vi "Launch Plugins.vi"(8 "error in":errorcluster, 11 "Master Controller in":refnum<class "EMS User Interface.lvclass">) -> (0 "error out":errorcluster, 3 "Master Controller out":refnum<class "EMS User Interface.lvclass">)   [LabVIEW 2018, in "EMS User Interface Actor.lvlib" / "EMS User Interface.lvclass"]
doc: "Launch SCADA. This nested actor handles all of the optimization and communication actors, so the Master Controller Core can focus on UI interaction."
uses:
  EMS User Interface.lvclass
  <vilib>/ActorFramework/Actor/Actor.lvclass
  EMS Generic Actor/EMS Generic/EMS Generic.lvclass
  C:/Users/Administrator/Desktop/2018LabVIEW EMS/EMS Generic Actor/EMS Generic/EMS Generic.lvclass
  C:/Program Files (x86)/National Instruments/LabVIEW 2018/vi.lib/ActorFramework/Actor/Actor.lvclass
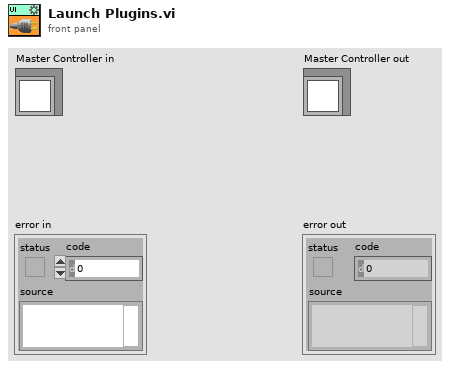
[diagram p1: front panel]
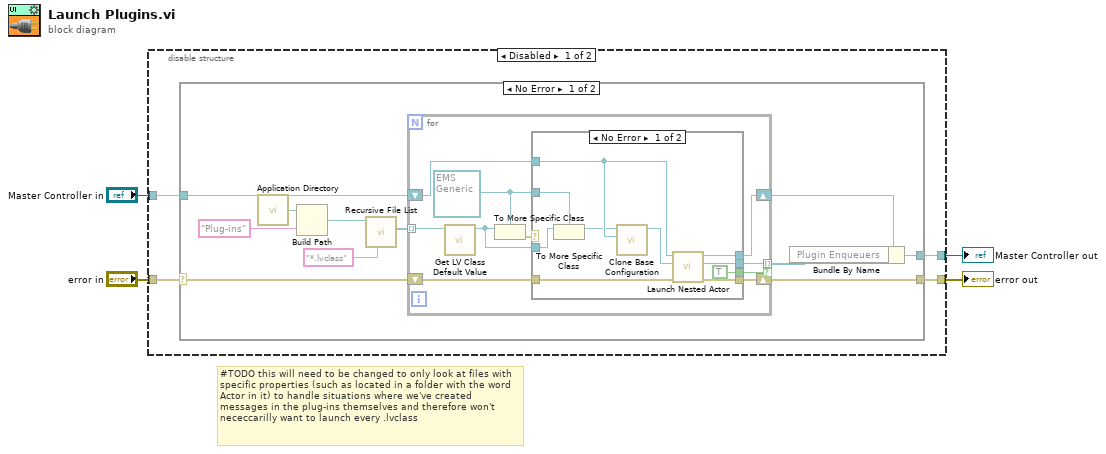
[diagram p0: block diagram]
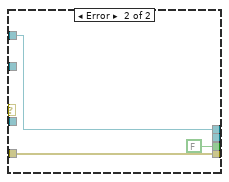
[diagram p2: hidden frame]
diagram:
  # "#TODO this will need to be changed to only look at files with specific properties (such as located in a folder with the word Actor in it) to handle situations where we've created messages in the plug-ins themselves and therefore won't nececcarilly want to launch every .lvclass"
  n1 = disable-structure shown="Disabled" {
    disable-tunnel: "error in" -> [w8 w45]
    disable-tunnel: [w7 w45] -> w3
    disable-tunnel: "Master Controller in" -> [w6 w46]
    disable-tunnel: [w5 w46] -> w1
    frame Disabled {
      n2 = case shown="No Error" w8 {
        selector: w8 -> [w16 w44]
        tunnel: [w17 w44] -> w7
        tunnel: [w18 w43] -> w5
        tunnel: w6 -> [w15 w43]
        frame No Error {
          n3 = call <vilib>:"Application Directory.vi"() -> ("Application Directory"=w10:path)
          n4 = Build Path(base path=w10, name or relative path="Plug-ins") -> (appended path=w12:path)
          n5 = call <vilib>:"Recursive File List.vi"("pattern"="*.lvclass", "Folder Path"=w12) -> ("All Files in Dir"=w9:path[])  [unwired: 5 in, 4 out]
          n6 = for {
            shift-right: [w28] -> w17
            shift-left: w16 -> [w27]
            shift-right: [w29] -> w19
            shift-left: w15 -> [w24]
            tunnel: [w26] -> w14 mode=indexing if=w21
            tunnel: w9 -> [w25] mode=indexing
            w22 = refnum<class "EMS Generic.lvclass"> refnum ("EMS Generic Actor.lvlib:EMS Generic.lvclass")
            n7 = call <vilib>:"Get LV Class Default Value.vi"("class path"=w25) -> ("object"=w20:refnum<class>)  [unwired: 9 in, 1 out]
            n8 = To More Specific Class(target class=w22, reference=w20) -> (error out=w23:errorcluster)  [unwired: 1 in, 1 out]
            n9 = case shown="No Error" w23 {
              tunnel: [w39 w42] -> w29
              tunnel: [w38 w40] -> w28
              tunnel: w27 -> [w37 w40]
              tunnel: [w36 _] -> w26
              tunnel: w24 -> [w34 w42]
              tunnel: w22 -> [w32 _]
              tunnel: [TRUE FALSE] -> w21
              tunnel: w20 -> [w30 _]
              frame No Error {
                n10 = To More Specific Class(target class=w32, reference=w30) -> (specific class reference=w33:refnum<class "EMS Generic.lvclass">)  [unwired: 1 in, 1 out]
                n11 = call-dynamic "Clone Base Configuration.vi"("Source Object"=w34, "Target Object in"=w33) -> ("Target Object out"=w35:refnum<class "EMS Generic.lvclass">)  [unwired: 9 in]
                n12 = call <vilib>:"Launch Nested Actor.vi"("error in (no error)"=w37, "Nested Actor"=w35, "Caller Actor in"=w34) -> ("error out"=w38:errorcluster, "Nested Actor's Enqueuer"=w36:refnum<class "Message Enqueuer.lvclass">, "Caller Actor out"=w39:refnum<class "EMS User Interface.lvclass">)  [unwired: 6 in]
              }
              frame Error {
              }
            }
          }
          n13 = Bundle By Name(cluster=w19, "Plugin Enqueuers"=w14) -> (w18:refnum<class "EMS User Interface.lvclass">)
        }
        frame Error {
        }
      }
    }
    frame Enabled {
    }
  }
  "error out" <- w3
  "Master Controller out" <- w1
